vi "Anaheim Open COM full loop.vi"(1 "MOTOR SELECTOR":dbl(knob)=1.0 min=0.0 max=10.0 step=1.0 scale=0.0..10.0 scale format="%#_2g", 3 "GO":bool, 5 "ACCEL/DECEL":dbl=8000.0, 7 "BASE SPEED":dbl=1000.0, 9 "MAX SPEED":dbl=10000.0, 11 "INDEX NUMBER":dbl=2000.0, 12 "COMPLETE TIME":dbl=3.0, 13 "PROGRAM PROFILE PARAMETERS":bool) -> ()   [LabVIEW 2018]
uses:
  9e8d34a8-7cf9-4e2b-a7b9-2bde2f7936eb.vi
  d6440aa1-291c-44ad-86aa-9318df412e43.vi
  e8f71ab3-fd59-4f70-99d8-18aca2006016.vi
  dfc31eb5-2ddb-4863-815f-2b9358a6c860.vi
  5ff84055-6964-4a11-80ad-64262a616194.vi
  <vilib>/Instr/_visa.llb/VISA Configure Serial Port (Serial Instr).vi
panel:
  in  "HALT":bool
  in  "Direction":bool=TRUE
  out "error code":u32
  in  "Clear Errors":bool
  in  "baud rate":u32=38400
  in  "stop bits (10: 1 bit)":u16(ring)=10 items=["1.0"=10, "1.5"=15, "2.0"=20]
  in  "VISA resource name":refnum<visa-resource-name>
  in  "stop":bool
  # "CCW"
  # "CW"
  # "(DISTANCE)"
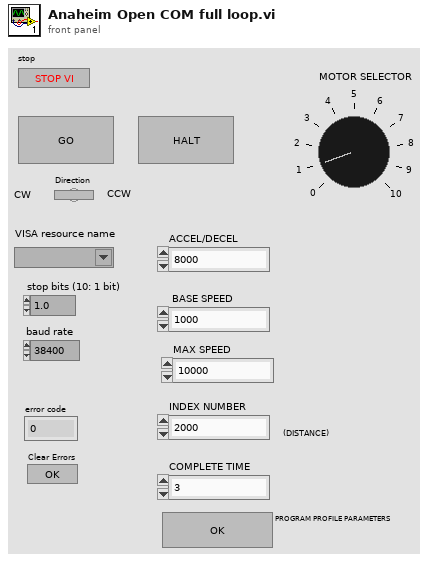
[diagram p1: front panel]
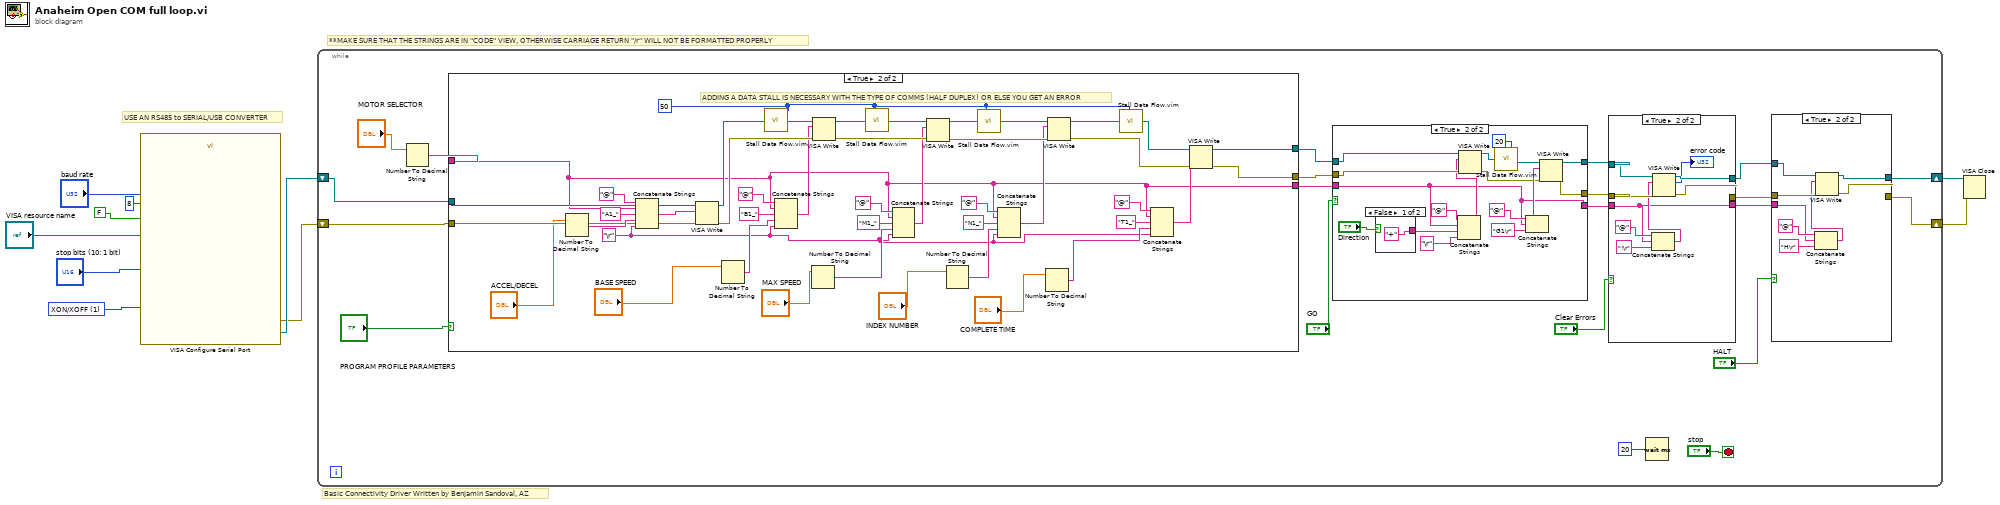
[diagram p0: block diagram]
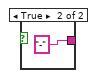
[diagram p6: hidden frame]
diagram:
  w6 = u16 1 items=["None", "XON/XOFF", "RTS/CTS", "XON/XOFF & RTS/CTS", "DTR/DSR", "XON/XOFF & DTR/DSR"] ("flow control (0:none)")
  # "Basic Connectivity Driver Written by Benjamin Sandoval, AZ"
  # "USE AN RS485 to SERIAL/USB CONVERTER"
  # "**MAKE SURE THAT THE STRINGS ARE IN \"CODE\" VIEW, OTHERWiSE CARRIAGE RETURN \"/r\" WILL NOT BE FORMATTED PROPERLY"
  n1 = call-poly "VISA Configure Serial Port"("VISA resource name"="VISA resource name", "Enable Termination\nChar (T)"=FALSE, "baud rate (9600)"="baud rate", "data bits (8)"=8, "stop bits (10: 1 bit)"="stop bits (10: 1 bit)", "flow control (0:none)"=w6) -> ("VISA resource name out"=w8:refnum<visa-resource-name>, "error out"=w7:errorcluster)  [unwired: 8 in]
  n2 = while {
    shift-right: [w13] -> w5
    shift-left: w8 -> [w22]
    shift-right: [w12] -> w1
    shift-left: w7 -> [w21]
    stop <- "stop" stop-if-true
    n3 = Number To Decimal String(number="MOTOR SELECTOR") -> (decimal integer string=w18:string)  [unwired: 1 in]
    n4 = case shown="True" "PROGRAM PROFILE PARAMETERS" {
      tunnel: w21 -> [w55 w96]
      tunnel: w22 -> [w56 w95]
      tunnel: [w56 w59] -> w28
      tunnel: [w55 w58] -> w27
      tunnel: [w54 w57] -> w20
      tunnel: w18 -> [w54 w57]
      frame False {
      }
      frame True {
        w60 = 50
        w77 = "\r"
        # "ADDING A DATA STALL IS NECESSARY WITH THE TYPE OF COMMS (HALF DUPLEX) OR ELSE YOU GET AN ERROR"
        n5 = Number To Decimal String(number="ACCEL/DECEL") -> (decimal integer string=w98:string)  [unwired: 1 in]
        n6 = Concatenate Strings("@", w57, "A1_", w98, w77) -> (w97:string)
        n7 = VISA Write(VISA resource name=w95, write buffer=w97, error in (no error)=w96) -> (VISA resource name out=w68:refnum<visa-resource-name>, error out=w76:errorcluster)  [unwired: 1 out]
        n8 = Number To Decimal String(number="BASE SPEED") -> (decimal integer string=w81:string)  [unwired: 1 in]
        n9 = call "Stall Data Flow.vim"("value in"=w68, "milliseconds to wait"=w60) -> ("value out"=w67:refnum<visa-resource-name>)  [unwired: 1 out]
        n10 = Concatenate Strings("@", w57, "B1_", w81, w77) -> (w75:string)
        n11 = Number To Decimal String(number="MAX SPEED") -> (decimal integer string=w80:string)  [unwired: 1 in]
        n12 = VISA Write(VISA resource name=w67, write buffer=w75, error in (no error)=w76) -> (VISA resource name out=w66:refnum<visa-resource-name>, error out=w74:errorcluster)  [unwired: 1 out]
        n13 = call "Stall Data Flow.vim"("value in"=w66, "milliseconds to wait"=w60) -> ("value out"=w65:refnum<visa-resource-name>)  [unwired: 1 out]
        n14 = Concatenate Strings("@", w57, "M1_", w80, w77) -> (w71:string)
        n15 = VISA Write(VISA resource name=w65, write buffer=w71, error in (no error)=w74) -> (VISA resource name out=w64:refnum<visa-resource-name>, error out=w73:errorcluster)  [unwired: 1 out]
        n16 = Number To Decimal String(number="INDEX NUMBER") -> (decimal integer string=w79:string)  [unwired: 1 in]
        n17 = call "Stall Data Flow.vim"("value in"=w64, "milliseconds to wait"=w60) -> ("value out"=w63:refnum<visa-resource-name>)  [unwired: 1 out]
        n18 = Concatenate Strings("@", w57, "N1_", w79, w77) -> (w70:string)
        n19 = Number To Decimal String(number="COMPLETE TIME") -> (decimal integer string=w78:string)  [unwired: 1 in]
        n20 = VISA Write(VISA resource name=w63, write buffer=w70, error in (no error)=w73) -> (VISA resource name out=w62:refnum<visa-resource-name>, error out=w72:errorcluster)  [unwired: 1 out]
        n21 = call "Stall Data Flow.vim"("value in"=w62, "milliseconds to wait"=w60) -> ("value out"=w61:refnum<visa-resource-name>)  [unwired: 1 out]
        n22 = Concatenate Strings("@", w57, "T1_", w78, w77) -> (w69:string)
        n23 = VISA Write(VISA resource name=w61, write buffer=w69, error in (no error)=w72) -> (VISA resource name out=w59:refnum<visa-resource-name>, error out=w58:errorcluster)  [unwired: 1 out]
      }
    }
    n24 = case shown="True" "GO" {
      tunnel: w28 -> [w103 w111]
      tunnel: w27 -> [w102 w109]
      tunnel: [w103 w120] -> w24
      tunnel: [w102 w119] -> w23
      tunnel: w20 -> [w101 w104]
      tunnel: [w101 w104] -> w17
      frame False {
      }
      frame True {
        n25 = case shown="False" "Direction" {
          tunnel: ["+" "-"] -> w112
          frame False {
          }
          frame True {
          }
        }
        n26 = Concatenate Strings("@", w104, w112, "\r") -> (w107:string)
        n27 = VISA Write(VISA resource name=w111, write buffer=w107, error in (no error)=w109) -> (VISA resource name out=w110:refnum<visa-resource-name>, error out=w108:errorcluster)  [unwired: 1 out]
        n28 = call "Stall Data Flow.vim"("value in"=w110, "milliseconds to wait"=20) -> ("value out"=w106:refnum<visa-resource-name>)  [unwired: 1 out]
        n29 = Concatenate Strings("@", w104, "G1\r") -> (w116:string)
        n30 = VISA Write(VISA resource name=w106, write buffer=w116, error in (no error)=w108) -> (VISA resource name out=w120:refnum<visa-resource-name>, error out=w119:errorcluster)  [unwired: 1 out]
      }
    }
    n31 = case shown="True" "Clear Errors" {
      tunnel: w24 -> [w44 w53]
      tunnel: [w44 w52] -> w16
      tunnel: w23 -> [w43 w51]
      tunnel: [w43 w50] -> w15
      tunnel: w17 -> [w42 w45]
      tunnel: [w42 w45] -> w14
      frame False {
      }
      frame True {
        n32 = Concatenate Strings("@", w45, "!\r") -> (w46:string)
        n33 = VISA Write(VISA resource name=w53, write buffer=w46, error in (no error)=w51) -> (VISA resource name out=w52:refnum<visa-resource-name>, return count=→"error code":u32, error out=w50:errorcluster)
      }
    }
    n34 = Wait (ms)(milliseconds to wait=20) -> ()  [unwired: 1 out]
    n35 = case shown="True" "HALT" {
      tunnel: w16 -> [w33 w41]
      tunnel: [w33 w40] -> w13
      tunnel: w15 -> [w32 w39]
      tunnel: [w32 w38] -> w12
      tunnel: w14 -> [_ w34]
      frame False {
      }
      frame True {
        n36 = Concatenate Strings("@", w34, "H\r") -> (w35:string)
        n37 = VISA Write(VISA resource name=w41, write buffer=w35, error in (no error)=w39) -> (VISA resource name out=w40:refnum<visa-resource-name>, error out=w38:errorcluster)  [unwired: 1 out]
      }
    }
  }
  n38 = VISA Close(VISA resource name=w5, error in (no error)=w1) -> ()  [unwired: 1 out]
